vi "get_number_of_devices.vi"(5 "error in (no error)":errorcluster, 7 "error dialog? (T)":bool=TRUE) -> (16 "num_of_devices (out)":i32, 19 "error out":errorcluster)   [LabVIEW 2020, in "classes.lvlib" / "_Controller.lvclass"]
doc: "Retrieve the number of identified USB Arcus devices.\n\nProduced By:\n\n<B>Kod Integrations, LLC</B>\n4835 Marianne Drive\nMount Airy, MD 21771\nhttp://www.kodintegrations.com\nemail: info@kodintegrations.com\nphone: (240) 687-1288"
uses:
  classes/Controller/_Controller.lvclass
  common/controls/error_actions.ctl
  PerformaxCom.dll
  libraries/common.lvlib
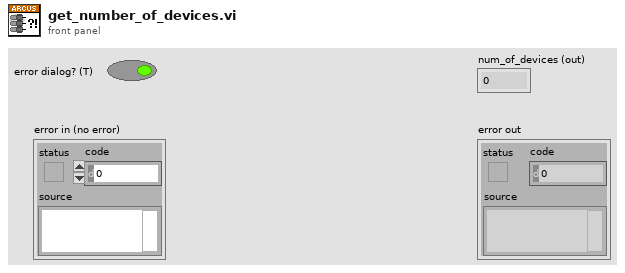
[diagram p1: front panel]
types:
  T1 = typedef "common.lvlib/error_actions.ctl" = enum16{"clearBuff", "closeRef", "nodeErr", "noDeviceInfo", "noDevices", "openRef", "sendReceive", "setTimeouts", "unknown"}
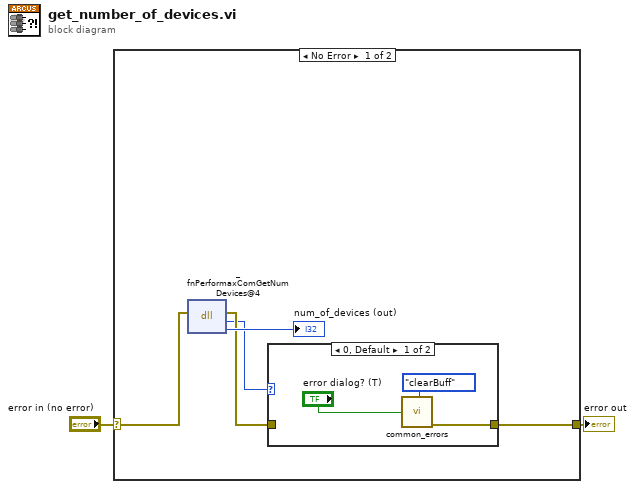
[diagram p0: block diagram]
diagram:
  n1 = case shown="No Error" "error in (no error)" {
    selector: "error in (no error)" -> [w3 w12]
    tunnel: [w4 w12] -> w1
    frame No Error {
      n2 = dll-call lib="PerformaxCom.dll" fn="_fnPerformaxComGetNumDevices@4"(error in=w3) -> (error out=w6:errorcluster, w5:i32, "numDevices"=→"num_of_devices (out)":i32)  [unwired: 3 in, 1 out]
      n3 = case shown="0, Default" w5 {
        tunnel: [w9 w11] -> w4
        tunnel: w6 -> [_ w11]
        frame 0, Default {
          n4 = call "common_errors.vi"("common_errors"=error_actions."clearBuff" ("errors"), "dialog? (T)"="error dialog? (T)") -> ("error out"=w9:errorcluster)  [unwired: 13 in]
        }
        frame 1 {
        }
      }
    }
    frame Error {
    }
  }
  "error out" <- w1
